vi "Lockin Engine.vi"(8 "error in (no error)":errorcluster, 9 "Reference":T3, 10 "AI Waveforms":waveform(dbl)[](array[waveform]), 11 "Lockin.DAQ":refnum<class "Lockin.DAQ.lvclass">) -> (0 "error out":errorcluster, 1 "SweepResults":T1, 2 "Averaged Results (X,Y,R,Theta,Mean)":T2 {"Results" format="%#_6p"}, 3 "Lockin.DAQ":refnum<class "Lockin.DAQ.lvclass">)   [LabVIEW 2016, in "Lockin.DAQ.lvclass"]
uses:
  Lockin.DAQ.lvclass
  Typedefs/Results--Cluster.ctl
  Typedefs/SweepResults--Cluster.ctl
  Lockin.DAQ.lvclass/Lockin.DAQ.ctl
  <vilib>/Analysis/baseanly.llb/Mean (DBL).vi
  <vilib>/Analysis/2dsp.llb/Decimate (single shot).vi
  <vilib>/Analysis/2dsp.llb/Decimate (single shot, DBL).vi
  <vilib>/Utility/High Resolution Relative Seconds.vi
  <vilib>/Waveform/WDTOps.llb/Number of Waveform Samples.vi
  <vilib>/Waveform/WDTOps.llb/WDT Number of Waveform Samples DBL.vi
  <vilib>/Utility/error.llb/Error Cluster From Error Code.vi
  <vilib>/Analysis/NI_AALBase.lvlib
panel:
  out "Y Results":cluster{i32[], dbl[]}[](graph)
  out "X Results":cluster{i32[], dbl[]}[](graph)
  out "filter fC (Hz)":dbl=0.3183098861837907
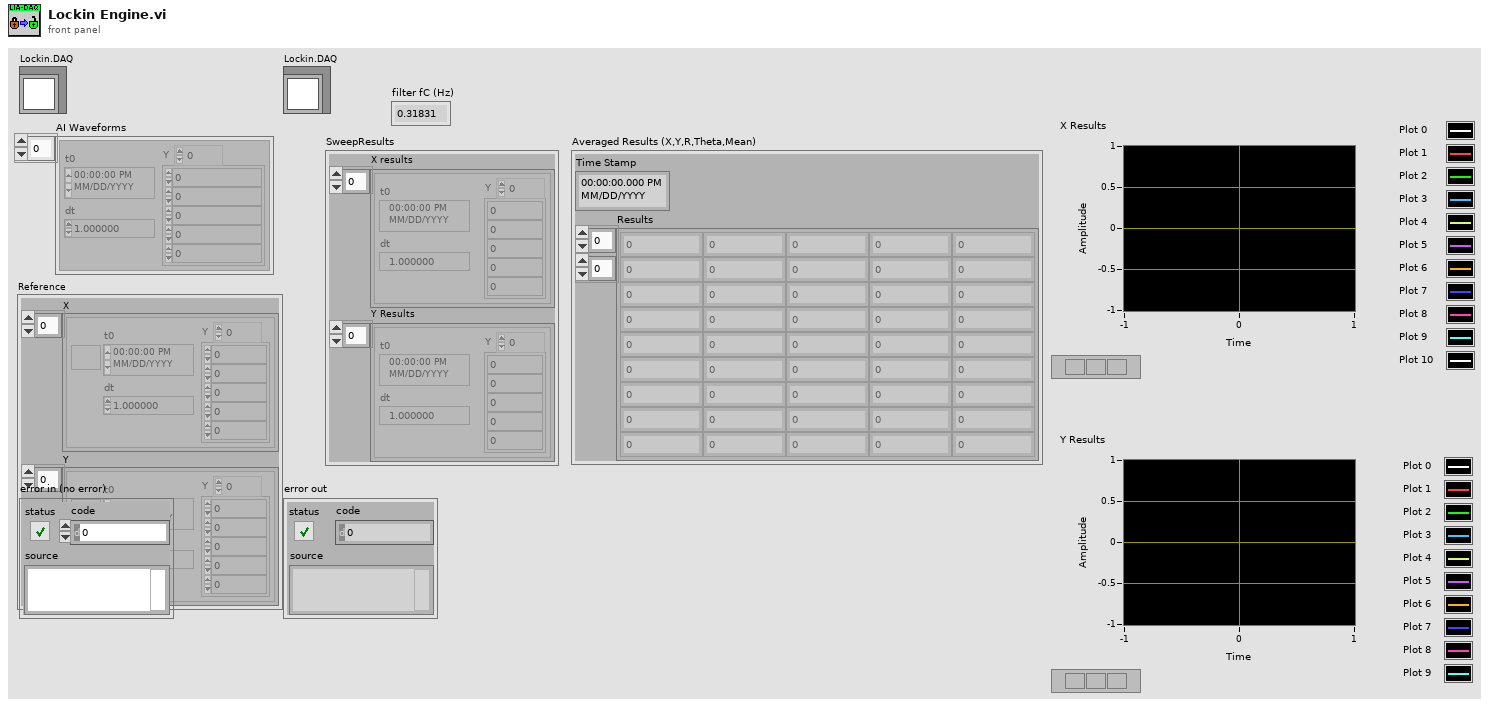
[diagram p1: front panel]
types:
  T1 = typedef "Lockin.DAQ.lvclass/SweepResults--Cluster.ctl" = cluster{"X results":waveform(dbl)[], "Y Results":waveform(dbl)[]}
  T2 = typedef "Lockin.DAQ.lvclass/Results--Cluster.ctl" = cluster{"Time Stamp":timestamp, "Results":dbl[][]}
  T3 = cluster{"X":waveform(dbl)[], "Y":waveform(dbl)[]}
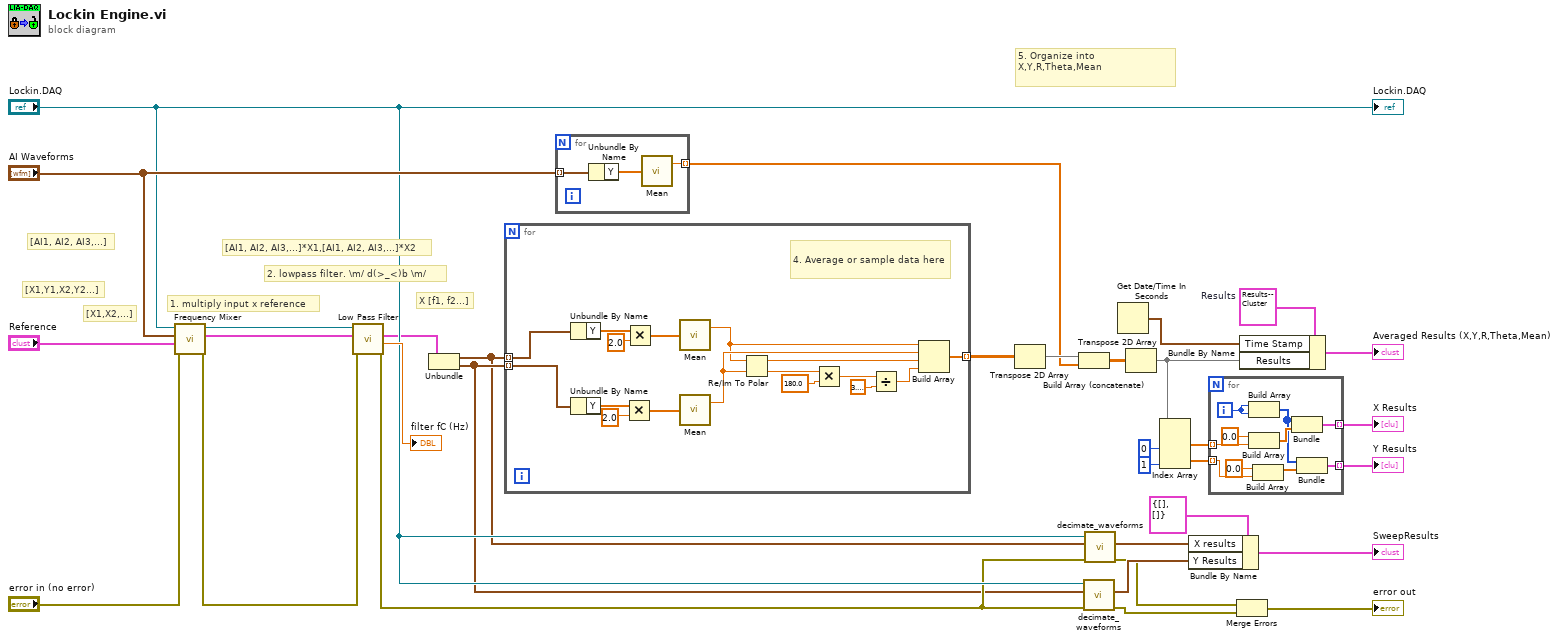
[diagram p0: block diagram]
diagram:
  w32 = T2 {"Time Stamp"=timestamp(0 s since 1904-01-01), "Results"=[]}  # Results
  # "[X1,X2,...]"
  # "1. multiply input x reference"
  # "X [f1, f2...]"
  # "2. lowpass filter. \\m/ d(>_<)b \\m/"
  # "[AI1, AI2, AI3,...]*X1,[AI1, AI2, AI3,...]*X2"
  # "[AI1, AI2, AI3,...]"
  # "[X1,Y1,X2,Y2...]"
  # "5. Organize into X,Y,R,Theta,Mean"
  n1 = call "Frequency Mixer.vi"("error in (no error)"="error in (no error)", "Reference"="Reference", "Signal []"="AI Waveforms", "Lockin.DAQ"="Lockin.DAQ") -> ("error out"=w6:errorcluster, "Mixed"=w7:T3, "Lockin.DAQ"=w18:refnum<class "Lockin.DAQ.lvclass">)  [unwired: 5 in]
  n2 = call "Low Pass Filter.vi"("error in (no error)"=w6, "Reference"=w7, "Lockin.DAQ"=w18) -> ("error out"=w5:errorcluster, "Fc (Hz)"=→"filter fC (Hz)":dbl, "Filtered"=w3:T3)  [unwired: 5 in, 1 out]
  n3 = Unbundle(w3) -> ("X"=w1:waveform(dbl)[], "Y"=w2:waveform(dbl)[])
  n4 = for {
    tunnel: [w44] -> w25 mode=indexing
    tunnel: w1 -> [w35] mode=indexing
    tunnel: w2 -> [w34] mode=indexing
    # "4. Average or sample data here"
    n5 = Unbundle By Name(w35) -> ("Y"=w42:dbl[])
    n6 = Unbundle By Name(w34) -> ("Y"=w40:dbl[])
    n7 = Multiply(x=w40, y=2.0) -> (x*y=w38:dbl[])
    n8 = Multiply(x=w42, y=2.0) -> (x*y=w39:dbl[])
    n9 = call-poly <vilib>:"Mean.vi"("X"=w39) -> ("mean"=w36:dbl)  [unwired: 1 out]
    n10 = call-poly <vilib>:"Mean.vi"("X"=w38) -> ("mean"=w37:dbl)  [unwired: 1 out]
    n11 = Re/Im To Polar(2:w37, 3:w36) -> (0:w47:dbl, 1:w45:dbl)
    n12 = Multiply(x=w47, y=180.0) -> (x*y=w46:dbl)
    n13 = Divide(x=w46, y=3.141592653589793) -> (x/y=w50:dbl)
    n14 = Build Array(w36, w37, w45, w50) -> (w44:dbl[])
  }
  n15 = for {
    tunnel: "AI Waveforms" -> [w52] mode=indexing
    tunnel: [w53] -> w19 mode=indexing
    n16 = Unbundle By Name(w52) -> ("Y"=w51:dbl[])
    n17 = call-poly <vilib>:"Mean.vi"("X"=w51) -> ("mean"=w53:dbl)  [unwired: 1 out]
  }
  n18 = Transpose 2D Array(2D array=w25) -> (transposed array=w33:dbl[][])
  n19 = Build Array (concatenate)(w33, w19) -> (w29:dbl[][])
  n20 = call "decimate_waveforms.vi"("error in (no error)"=w5, "WFM"=w2, "LockinDAQ"="Lockin.DAQ") -> ("error out"=w10:errorcluster, "WFM out"=w12:waveform(dbl)[])  [unwired: 6 in, 1 out]
  n21 = call "decimate_waveforms.vi"("error in (no error)"=w5, "WFM"=w1, "LockinDAQ"="Lockin.DAQ") -> ("error out"=w9:errorcluster, "WFM out"=w13:waveform(dbl)[])  [unwired: 6 in, 1 out]
  n22 = Get Date/Time In Seconds() -> (seconds since 1Jan1904=w31:timestamp)
  n23 = Transpose 2D Array(2D array=w29) -> (transposed array=w27:dbl[][])
  n24 = Index Array(array=w27, index (col) #1=0 ("disabled index (col)"), index (col) #2=1 ("index (col)")) -> (element #1=w28:dbl[], element #2=w22:dbl[])  [unwired: 2 in]
  n25 = Bundle By Name(cluster=T1 {"X results"=[], "Y Results"=[]} ("SweepResults"), "X results"=w13, "Y Results"=w12) -> (→"SweepResults":T1)
  n26 = for {
    tunnel: w28 -> [w63] mode=indexing
    tunnel: [w61] -> w26 mode=indexing
    tunnel: w22 -> [w55] mode=indexing
    tunnel: [w54] -> w21 mode=indexing
    i -> [w60]
    n27 = Build Array(w60, w60) -> (w57:i32[])
    n28 = Build Array(0.0 ("element"), w63) -> (w59:dbl[])
    n29 = Build Array(0.0 ("element"), w55) -> (w56:dbl[])
    n30 = Bundle(w57, w59) -> (w61:cluster{i32[], dbl[]})  [unwired: 1 in]
    n31 = Bundle(w57, w56) -> (w54:cluster{i32[], dbl[]})  [unwired: 1 in]
  }
  "X Results" <- w26
  "Y Results" <- w21
  n32 = Merge Errors(w9, w10) -> (→"error out":errorcluster)
  n33 = Bundle By Name(cluster=w32, "Time Stamp"=w31, "Results"=w27) -> (→"Averaged Results (X,Y,R,Theta,Mean)":T2)
  "Lockin.DAQ" <- "Lockin.DAQ"
